vi "Move.vi"(8 "error in (no error)":errorcluster, 9 "Current XYZ Position":T3 {"Z" format="Z= %#_g"; "Y" format="Y= %#_g"; "X" format="X= %#_g"}, 10 "XYZ Position Input":T1={"Speed"=0, "Z Limit (um+/-)"=0.0, "Axes"="Z", "XYZ Coordinates"={"X"=0.0, "Y"=0.0, "Z"=0.0}} {"XYZ Coordinates"."Z" format="Z= %#_g"; "XYZ Coordinates"."Y" format="Y= %#_g"; "XYZ Coordinates"."X" format="X= %#_g"; "Z Limit (um+/-)" format="Z Limit = %.0f"; "Speed" format="Speed= %.0f"}, 11 "Scientifica XYZ Gen1 in":refnum<class "Scientifica XYZ Gen1.lvclass">) -> (0 "error out":errorcluster, 2 "XYZ Position Command Output":T1={"Speed"=0, "Z Limit (um+/-)"=0.0, "Axes"="All", "XYZ Coordinates"={"X"=0.0, "Y"=0.0, "Z"=0.0}} {"XYZ Coordinates"."Z" format="Z= %#_g"; "XYZ Coordinates"."Y" format="Y= %#_g"; "XYZ Coordinates"."X" format="X= %#_g"; "Z Limit (um+/-)" format="Z Limit = %.0f"; "Speed" format="Speed= %.0f"}, 3 "Scientifica XYZ Gen1 out":refnum<class "Scientifica XYZ Gen1.lvclass">)   [LabVIEW 2020, in "TranslationStageClassStructure.lvlib" / "Scientifica XYZ Gen1.lvclass"]
uses:
  Scientifica XYZ Gen1.lvclass
  XYZ Stage Control/typedefs/XYZ_position_input.ctl
  XYZ Stage Control/typedefs/XYZ axes.ctl
  Typedefs/XYZ_coordinates.ctl
  Scientifica XYZ Gen1.lvclass/Scientifica XYZ Gen1.ctl
  Serial Comms/Serial Comms/Serial Comms.lvclass
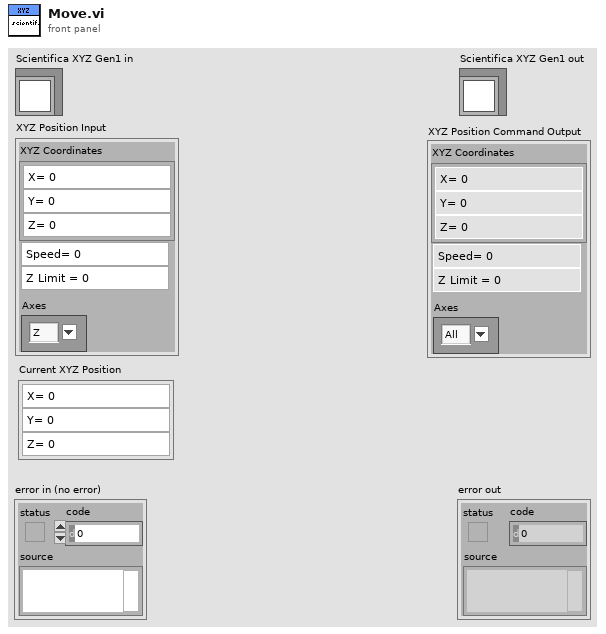
[diagram p1: front panel]
types:
  T1 = typedef "XYZ_position_input.ctl" = cluster{"Speed":i32, "Z Limit (um+/-)":sgl, "Axes":T2, "XYZ Coordinates":T3}
  T2 = typedef "XYZ axes.ctl" = string
  T3 = typedef "XYZ_coordinates.ctl" = cluster{"X":sgl, "Y":sgl, "Z":sgl}
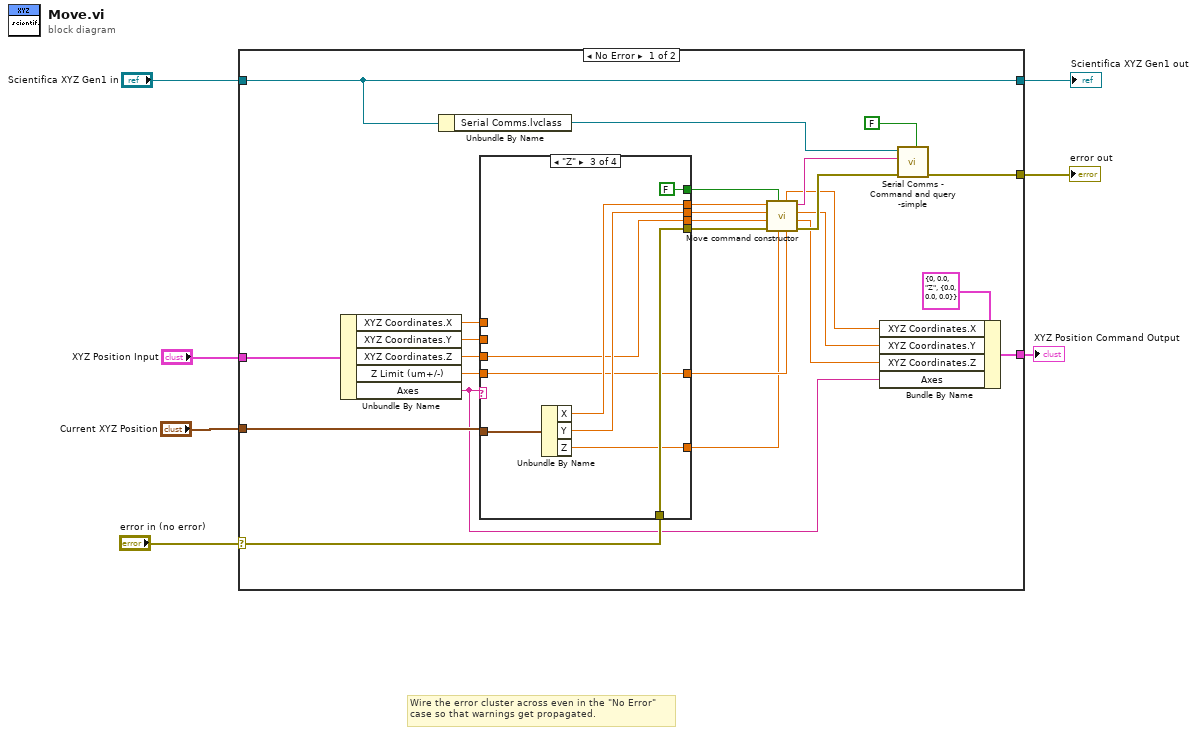
[diagram p0: block diagram]
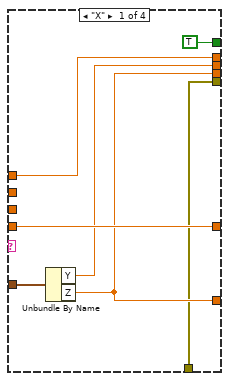
[diagram p2: hidden frame]
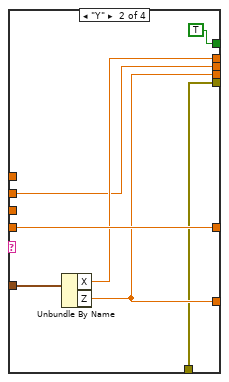
[diagram p3: hidden frame]
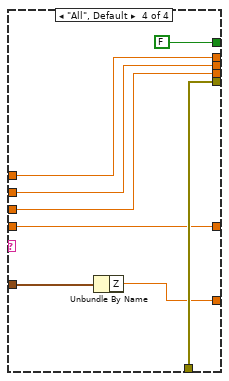
[diagram p4: hidden frame]
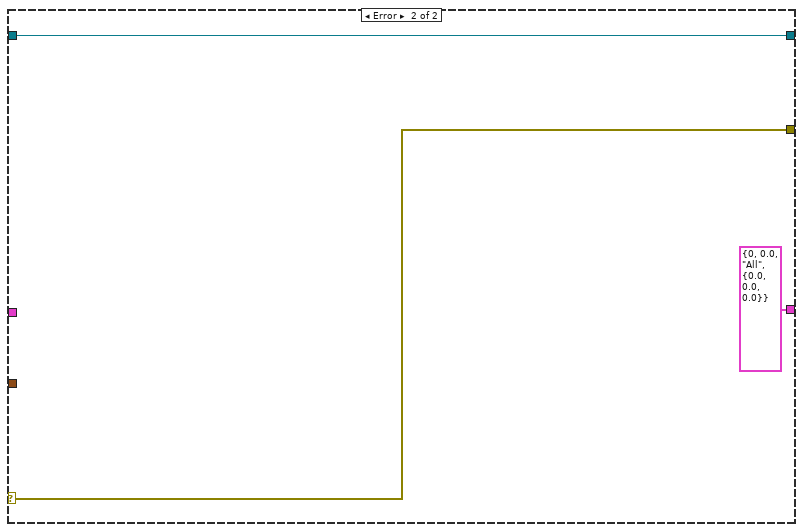
[diagram p5: hidden frame]
diagram:
  # "Wire the error cluster across even in the \"No Error\"\ncase so that warnings get propagated."
  n1 = case shown="No Error" "error in (no error)" {
    selector: "error in (no error)" -> [w29 w66]
    tunnel: [w24 w66] -> w6
    tunnel: [w32 w65] -> w4
    tunnel: "Scientifica XYZ Gen1 in" -> [w32 w65]
    tunnel: "XYZ Position Input" -> [w33 _]
    tunnel: "Current XYZ Position" -> [w14 _]
    tunnel: [w10 T1 {"Speed"=0, "Z Limit (um+/-)"=0.0, "Axes"="All", "XYZ Coordinates"={"X"=0.0, "Y"=0.0, "Z"=0.0}} ("XYZ Position Input 2")] -> w1
    frame No Error {
      n2 = Unbundle By Name(w33) -> ("XYZ Coordinates.X"=w28:sgl, "XYZ Coordinates.Y"=w27:sgl, "XYZ Coordinates.Z"=w26:sgl, "Z Limit (um+/-)"=w25:sgl, "Axes"=w8:T2)
      n3 = Unbundle By Name(w32) -> ("Serial Comms.lvclass"=w31:refnum<class "Serial Comms.lvclass">)
      n4 = case shown="\"Z\"" w8 {
        tunnel: w29 -> [w35 w42 w51 w63]
        tunnel: w28 -> [w38 _ _ w62]
        tunnel: w27 -> [_ w44 _ w61]
        tunnel: w26 -> [_ _ w52 w60]
        tunnel: w25 -> [w39 w46 w50 w58]
        tunnel: [w35 w42 w51 w63] -> w23
        tunnel: [w38 w45 w54 w62] -> w21
        tunnel: [w37 w44 w53 w61] -> w20
        tunnel: [w36 w43 w52 w60] -> w19
        tunnel: [TRUE ("Bypass Z-safety interlock") TRUE ("Bypass Z-safety interlock") FALSE ("Bypass Z-safety interlock") FALSE ("Bypass Z-safety interlock")] -> w17
        tunnel: [w39 w46 w50 w58] -> w16
        tunnel: w14 -> [w40 w47 w55 w57]
        tunnel: [w36 w43 w48 w56] -> w15
        frame "X" {
          n5 = Unbundle By Name(w40) -> ("Y"=w37:sgl, "Z"=w36:sgl)
        }
        frame "Y" {
          n6 = Unbundle By Name(w47) -> ("X"=w45:sgl, "Z"=w43:sgl)
        }
        frame "Z" {
          n7 = Unbundle By Name(w55) -> ("X"=w54:sgl, "Y"=w53:sgl, "Z"=w48:sgl)
        }
        frame "All", Default {
          n8 = Unbundle By Name(w57) -> ("Z"=w56:sgl)
        }
      }
      n9 = call "Move command constructor.vi"("Z Limit (+/- um)"=w16, "Z Current"=w15, "Bypass Z-safety interlock"=w17, "error in (no error)"=w23, "Z"=w19, "Y"=w20, "X"=w21) -> ("error out"=w22:errorcluster, "Adjusted Z"=w11:sgl, "Adjusted Y"=w12:sgl, "Move command"=w18:string, "Adjusted X"=w13:sgl)
      n10 = Bundle By Name(cluster=T1 {"Speed"=0, "Z Limit (um+/-)"=0.0, "Axes"="Z", "XYZ Coordinates"={"X"=0.0, "Y"=0.0, "Z"=0.0}} ("XYZ Position Input 2"), "XYZ Coordinates.X"=w13, "XYZ Coordinates.Y"=w12, "XYZ Coordinates.Z"=w11, "Axes"=w8) -> (w10:T1)
      n11 = call "Serial Comms - Command and query -simple.vi"("Read response? (T)"=FALSE, "error in (no error)"=w22, "string to write"=w18, "Serial Comms in"=w31) -> ("error out"=w24:errorcluster)  [unwired: 3 in, 4 out]
    }
    frame Error {
    }
  }
  "error out" <- w6
  "Scientifica XYZ Gen1 out" <- w4
  "XYZ Position Command Output" <- w1
